vi "CT-Globals.vi"() -> ()   [LabVIEW 2015]
panel:
  in  "LUT":dbl[](array[numeric])
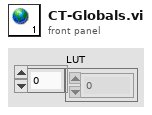
[diagram p1: front panel]
diagram:
